vi "Reference.vi"() -> ()   [LabVIEW 2009]
panel:
  out "Reference":i32
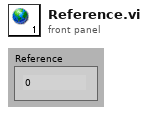
[diagram p1: front panel]
diagram:
